vi "AddToActiveProject.vi"(8 "error in (no error)":errorcluster, 11 "FlexUIActorMaker in":refnum<class "FlexUIActorMaker.lvclass">) -> (0 "error out":errorcluster, 3 "FlexUIActorMaker out":refnum<class "FlexUIActorMaker.lvclass">)   [LabVIEW 2016, in "FlexUIActorMaker.lvlib" / "FlexUIActorMaker.lvclass"]
uses:
  FlexUIActorMaker.lvclass
  FlexUIActorMaker.lvclass/FlexUIActorMaker.ctl
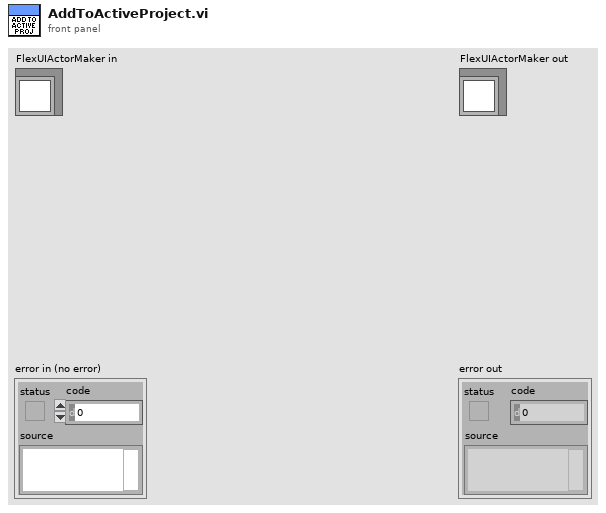
[diagram p1: front panel]
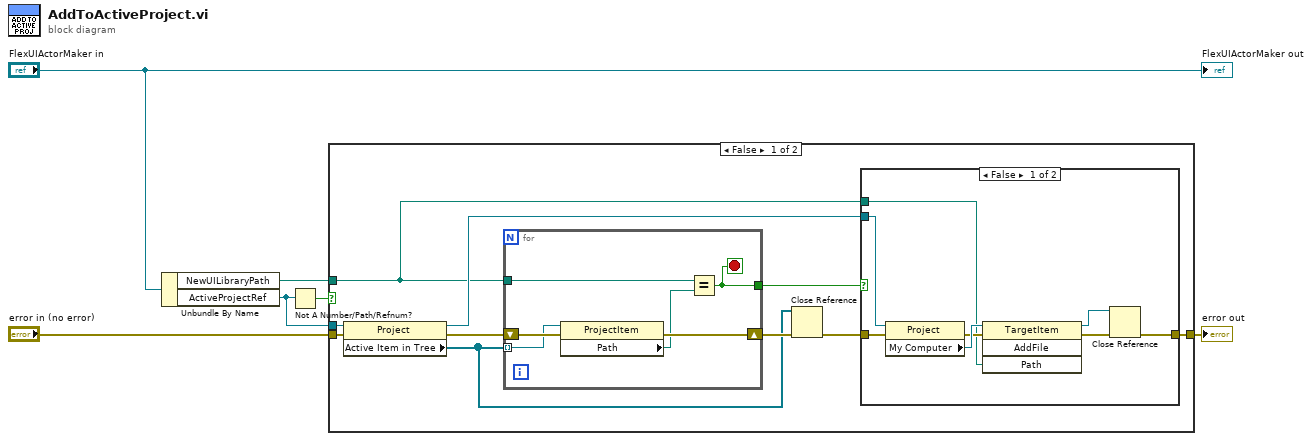
[diagram p0: block diagram]
diagram:
  n1 = Unbundle By Name("FlexUIActorMaker in") -> ("NewUILibraryPath"=w3:path, "ActiveProjectRef"=w2:refnum<vi>)
  n2 = Not A Number/Path/Refnum?(number/path/refnum=w2) -> (NaN/Path/Refnum?=w1:bool)
  n3 = case shown="False" w1 {
    tunnel: "error in (no error)" -> [w16 w32]
    tunnel: [w13 w32] -> w4
    tunnel: w3 -> [w8 _]
    tunnel: w2 -> [w7 _]
    frame False {
      n4 = property class="Project"(reference=w7, error in=w16) -> (reference out=w9:refnum<vi>, error out=w15:errorcluster, "Active Item in Tree"=w10:refnum<vi>[])
      n5 = for {
        shift-right: [w30] -> w12
        shift-left: w15 -> [w31]
        tunnel: w10 -> [w29] mode=indexing
        tunnel: w8 -> [w27]
        tunnel: [w26] -> w14
        stop <- w26 stop-if-true
        n6 = property class="ProjectItem"(reference=w29, error in=w31) -> (error out=w30:errorcluster, "Path"=w28:path)  [unwired: 1 out]
        n7 = Equal?(x=w27, y=w28) -> (x = y?=w26:bool)
      }
      n8 = Close Reference(reference=w10, error in (no error)=w12) -> (error out=w11:errorcluster)
      n9 = case shown="False" w14 {
        tunnel: [w18 w25] -> w13
        tunnel: w11 -> [w23 w25]
        tunnel: w9 -> [w24 _]
        tunnel: w8 -> [w20 _]
        frame False {
          n10 = property class="Project"(reference=w24, error in=w23) -> (error out=w21:errorcluster, "My Computer"=w22:refnum<vi>)  [unwired: 1 out]
          n11 = invoke class="TargetItem" method="AddFile"(reference=w22, error in=w21, "Path"=w20) -> (reference out=w17:refnum<vi>, error out=w19:errorcluster)  [unwired: 1 in, 2 out]
          n12 = Close Reference(reference=w17, error in (no error)=w19) -> (error out=w18:errorcluster)
        }
        frame True {
          # "Class already added to project."
        }
      }
    }
    frame True {
    }
  }
  "error out" <- w4
  "FlexUIActorMaker out" <- "FlexUIActorMaker in"
